vi "Read Single Digital In.vi"(6 "Value to Read":u32, 8 "error in":errorcluster, 11 "DIG_IO in":refnum<class "DIG_IO.lvclass">) -> (0 "error out":errorcluster, 2 "Value":bool, 3 "DIG_IO out":refnum<class "DIG_IO.lvclass">)   [LabVIEW 2019, in "DIG_IO.lvlib" / "DIG_IO.lvclass"]
doc: "This routine reads a specific digital input.\n\nThe value in is a U32 which is the largest typdef size available. This allows end development to have typdef enums mapped to the digital output pins creating human readable code."
uses:
  Library/DIG_IO.lvclass
  Library/DIG_IO.lvclass/DIG_IO.ctl
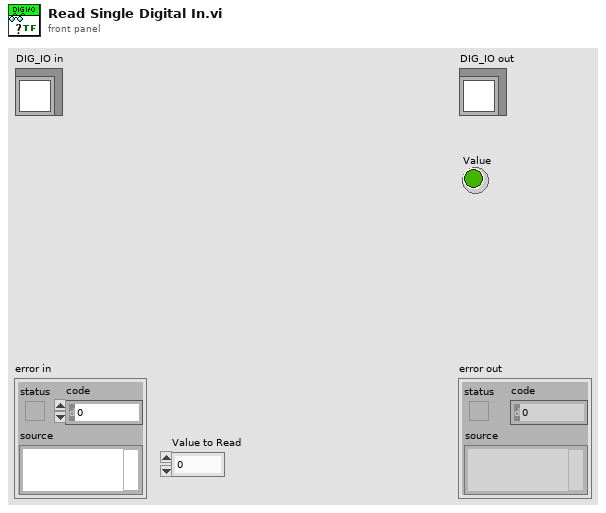
[diagram p1: front panel]
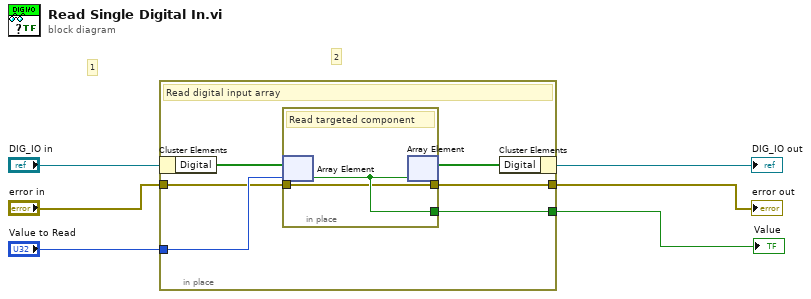
[diagram p0: block diagram]
diagram:
  # "2"
  # "1"
  n1 = in-place {
    in-place-border: [w11] -> w1
    in-place-border: "Value to Read" -> [w9]
    in-place-border: "error in" -> [w8]
    in-place-border: [w7] -> w2
    # "Read digital input array"
    n2 = in-place-cluster #1("DIG_IO in") -> ("Digital"=w12:bool[])
    n3 = in-place {
      in-place-border: [w14] -> w11
      in-place-border: w8 -> [w13]
      in-place-border: [w13] -> w7
      # "Read targeted component"
      n4 = in-place-array #2(w12, w9) -> (w14:bool)
      n5 = in-place-array #2(w14) -> (w10:bool[])  [unwired: 1 out]
    }
    n6 = in-place-cluster #1("Digital"=w10) -> (→"DIG_IO out":refnum<class "DIG_IO.lvclass">)
  }
  "error out" <- w2
  "Value" <- w1
